vi "Host_AutoApproach(Original).vi"() -> ()   [LabVIEW 2014]
uses:
  <vilib>/userdefined/High Color/nirio_resource_hc.ctl
  <vilib>/Instr/_visa.llb/VISA Configure Serial Port (Instr).vi
  <vilib>/FPGAPlugInAG/PCIe-7851R/niLvFpga_Open_PCIe-7851R.vi
  <vilib>/rvi/interface/common/dynamic/niFpgaDynamicAddResources.vi
  <vilib>/FPGAPlugInAG/Dynamic/niLvFpga_Run_Dynamic.vi
  <vilib>/Utility/error.llb/Error Cluster From Error Code.vi
  <vilib>/rvi/errors/niLvFpgaAdjustHostInterfaceError.vi
  <vilib>/FPGAPlugInAG/Dynamic/niLvFpga_Close_Dynamic.vi
  <vilib>/rvi/interface/nirviOpenFPGA/nirviOpenFPGA.xnode
  XZFPGAWithinHopping(Original)/FPGA Bitfiles/XZFPGAWithinHopp_FPGATarget_ApproachingStep(_p7iJPTKslXo.lvbitx
  <vilib>/rvi/interface/nirviMethod/nirviMethod.xnode
  <vilib>/rvi/interface/nirviReadWriteControl/nirviReadWriteControl.xnode
  <vilib>/rvi/interface/nirviCloseFPGA/nirviCloseFPGA.xnode
  NiFpgaLv.dll
  <vilib>/rvi/interface/Simulation/niFpgaSimulationCallBeginRW.vi
panel:
  out "ZCalPos":i32
  in  "PIZ":T1
  in  "ContinuousReapproach":bool
  in  "UseMemoryPos?":bool=TRUE
  out "ZRealPos":i16
  out "Curr":i16
  out "PIZPosDia":i16(graph)
  out "CurrDia":i16(graph)
  in  "stop":bool
  out "RoughZPos?":dbl
  out "Error?":string
  in  "RoughZ":refnum<visa-resource-name>
  in  "RoughZInitPos":dbl format="%#_13g"
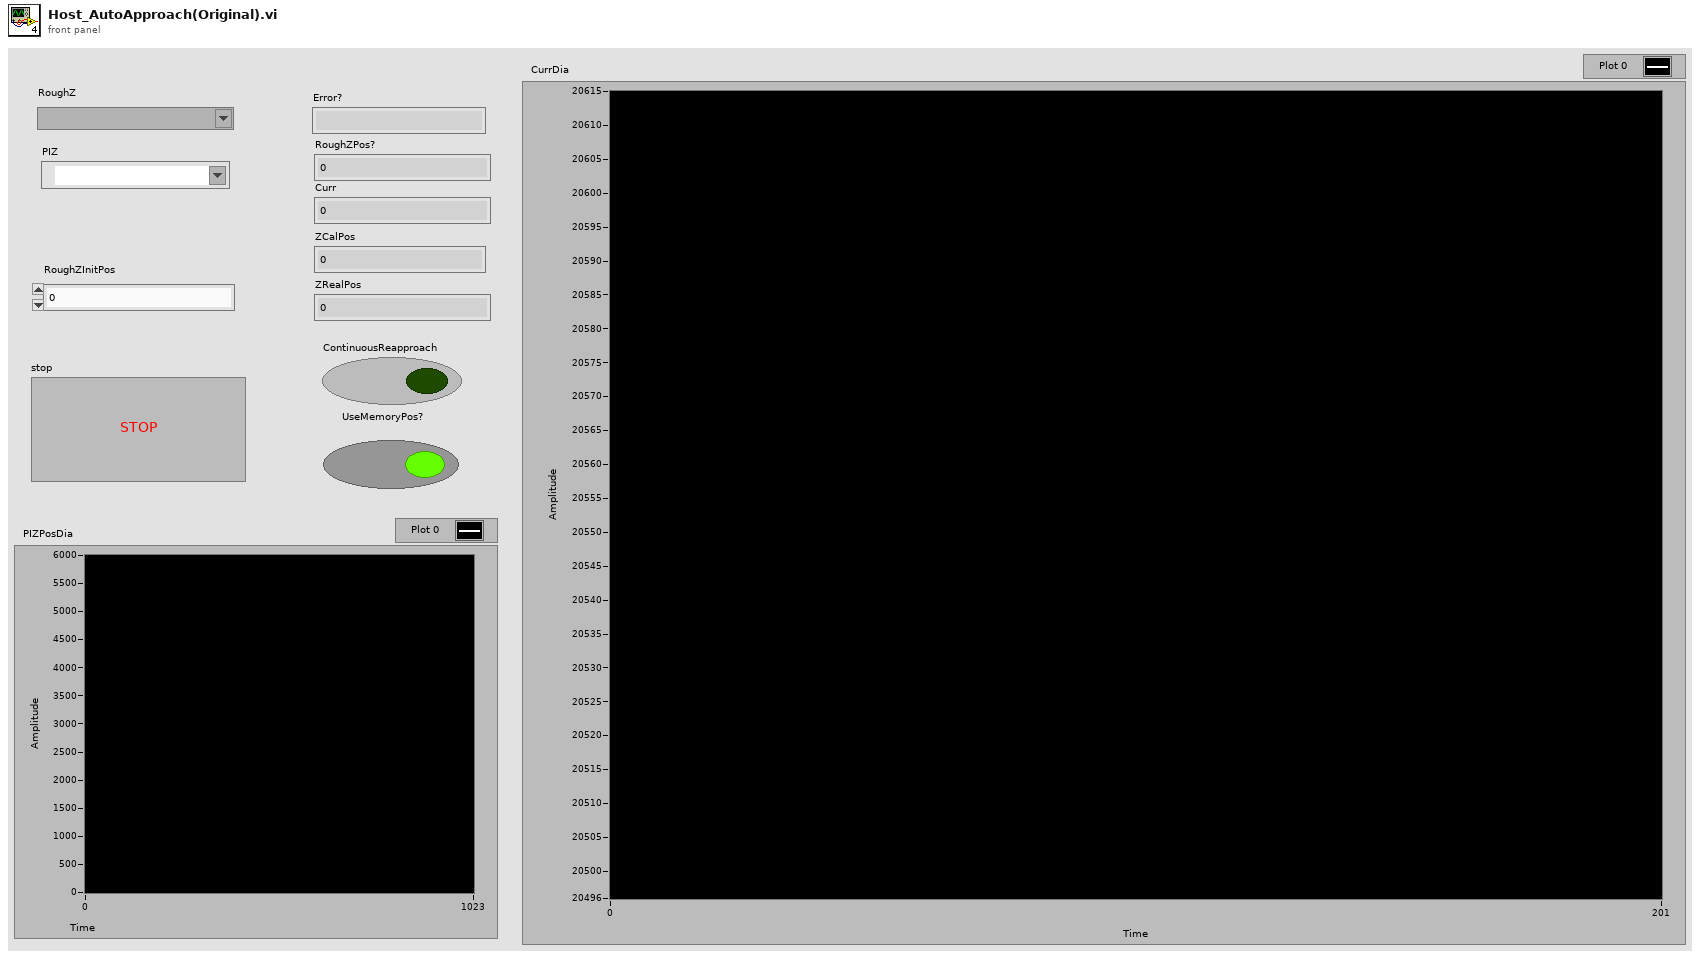
[diagram p1: front panel]
types:
  T1 = typedef "nirio_resource_hc.ctl" = tag
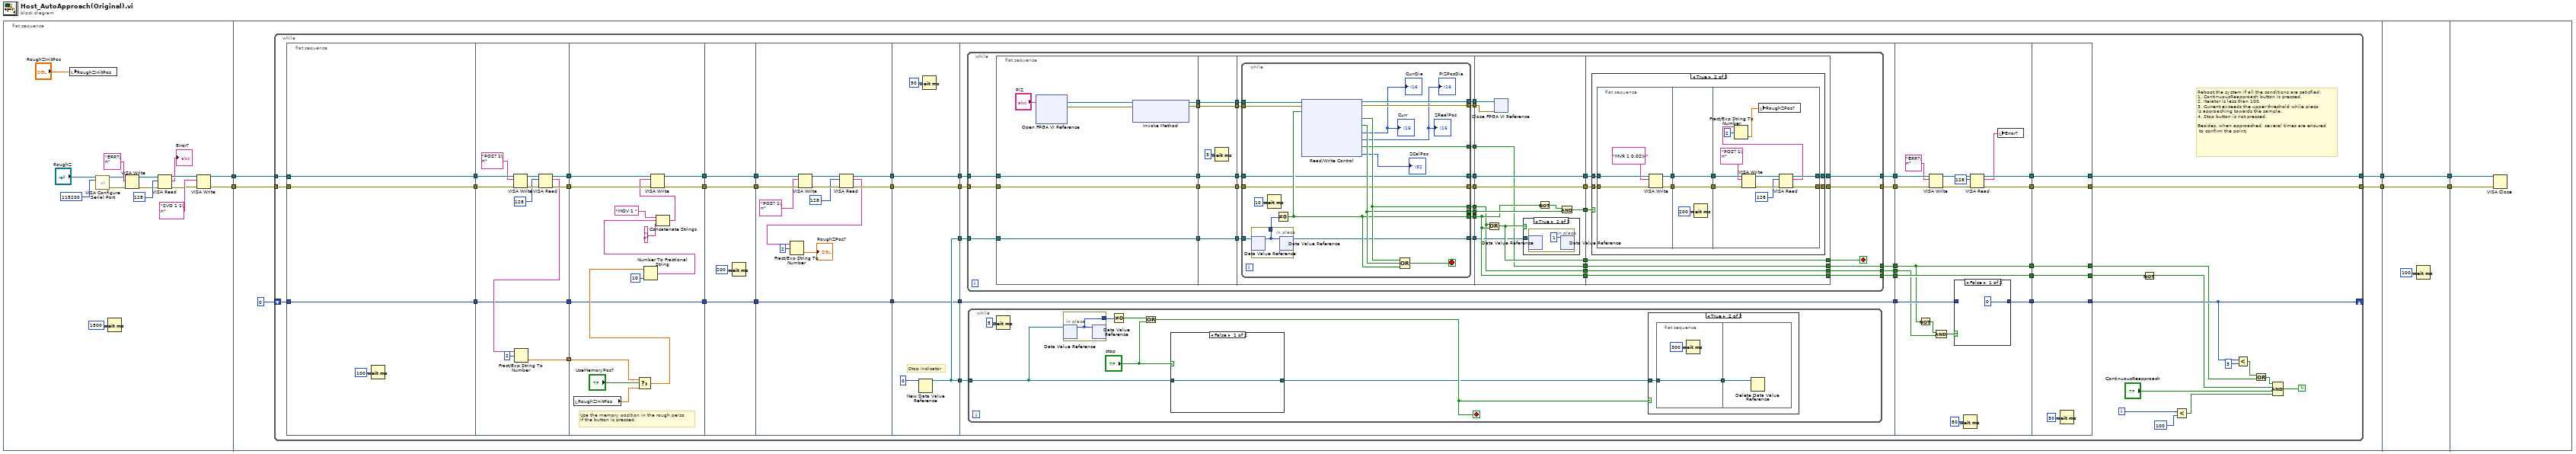
[diagram p0: block diagram]
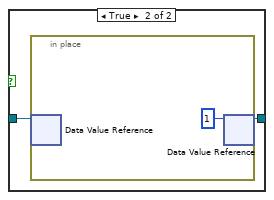
[diagram p3: hidden frame]
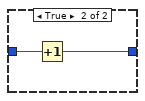
[diagram p6: hidden frame]
diagram:
  n1 = flat-sequence {
    tunnel: [w8] -> w2
    tunnel: [w7] -> w1
    tunnel: [w26] -> w5
    tunnel: [w25] -> w3
    tunnel: w2 -> [w24]
    tunnel: w1 -> [w23]
    tunnel: [w318] -> w6
    tunnel: w5 -> [w318]
    tunnel: [w317] -> w4
    tunnel: w3 -> [w317]
    tunnel: w6 -> [w320]
    tunnel: w4 -> [w319]
    frame #0 {
      n2 = local write "RoughZInitPos"("RoughZInitPos") -> ()
      n3 = call-poly "VISA Configure Serial Port"("VISA resource name"="RoughZ", "baud rate (9600)"=u32 115200) -> ("VISA resource name out"=w11:refnum<visa-resource-name>, "error out"=w12:errorcluster)  [unwired: 12 in]
      n4 = Wait (ms)(milliseconds to wait=u32 1500) -> ()  [unwired: 1 out]
      n5 = VISA Write(VISA resource name=w11, write buffer="ERR?\n", error in (no error)=w12) -> (VISA resource name out=w14:refnum<visa-resource-name>, error out=w15:errorcluster)  [unwired: 1 out]
      n6 = VISA Read(VISA resource name=w14, byte count=u32 128, error in (no error)=w15) -> (VISA resource name out=w18:refnum<visa-resource-name>, read buffer=→"Error?":string, error out=w19:errorcluster)  [unwired: 1 out]
      n7 = VISA Write(VISA resource name=w18, write buffer="SVO 1 1\n", error in (no error)=w19) -> (VISA resource name out=w8:refnum<visa-resource-name>, error out=w7:errorcluster)  [unwired: 1 out]
    }
    frame #1 {
      n8 = while {
        shift-right: [w36] -> _
        shift-left: 0 -> [w46]
        tunnel: [w31] -> w26
        tunnel: [w30] -> w25
        tunnel: w24 -> [w29]
        tunnel: w23 -> [w28]
        i -> [w57]
        stop <- w51 continue-if-true
        # "Reboot the system if all the conditions are satisfied:\n1. ContinuousReapproach button is pressed.\n2. Iterator is less than 100.\n3. Current exceeds the upper threshold while piezo\nis approaching towards the sample.\n4. Stop button is not pressed.\n\nBesides, when approached, several times are ensured\n to confirm the point."
        n9 = flat-sequence {
          tunnel: [w78] -> w76
          tunnel: [w77] -> w75
          tunnel: w46 -> [w80]
          tunnel: [w80] -> w45
          tunnel: w29 -> [w78]
          tunnel: w28 -> [w77]
          tunnel: w76 -> [w92]
          tunnel: [w88] -> w74
          tunnel: w75 -> [w91]
          tunnel: [w87] -> w73
          tunnel: [w82] -> w72
          tunnel: w45 -> [w81]
          tunnel: [w81] -> w44
          tunnel: w74 -> [w106]
          tunnel: w73 -> [w105]
          tunnel: [w99] -> w71
          tunnel: [w98] -> w70
          tunnel: w72 -> [w96]
          tunnel: w44 -> [w93]
          tunnel: [w93] -> w41
          tunnel: w71 -> [w110]
          tunnel: w70 -> [w109]
          tunnel: [w110] -> w69
          tunnel: [w109] -> w68
          tunnel: [w107] -> w42
          tunnel: w41 -> [w107]
          tunnel: w69 -> [w122]
          tunnel: w68 -> [w121]
          tunnel: [w116] -> w67
          tunnel: [w115] -> w66
          tunnel: [w111] -> w43
          tunnel: w42 -> [w111]
          tunnel: [w128] -> w65
          tunnel: [w127] -> w64
          tunnel: [w124] -> w63
          tunnel: [w124] -> w62
          tunnel: w66 -> [w127]
          tunnel: w67 -> [w128]
          tunnel: w43 -> [w123]
          tunnel: [w123] -> w40
          tunnel: w65 -> [w138]
          tunnel: w64 -> [w137]
          tunnel: w63 -> [w136]
          tunnel: w62 -> [w135]
          tunnel: [w134] -> w61
          tunnel: [w133] -> w60
          tunnel: [w132] -> w55
          tunnel: [w131] -> w50
          tunnel: w40 -> [w130]
          tunnel: [w130] -> w39
          tunnel: [w129] -> w38
          tunnel: w61 -> [w306]
          tunnel: w60 -> [w305]
          tunnel: [w300] -> w59
          tunnel: [w299] -> w58
          tunnel: w55 -> [w295]
          tunnel: [w295] -> w54
          tunnel: w50 -> [w292]
          tunnel: [w292] -> w49
          tunnel: w39 -> [w296]
          tunnel: w38 -> [w290]
          tunnel: [w293] -> w37
          tunnel: [w314] -> w48
          tunnel: [w313] -> w33
          tunnel: [w312] -> w31
          tunnel: [w311] -> w30
          tunnel: w49 -> [w313]
          tunnel: w54 -> [w314]
          tunnel: w58 -> [w311]
          tunnel: w59 -> [w312]
          tunnel: w37 -> [w310]
          tunnel: [w310] -> w36
          frame #0 {
            n10 = Wait (ms)(milliseconds to wait=u32 100) -> ()  [unwired: 1 out]
          }
          frame #1 {
            n11 = VISA Write(VISA resource name=w92, write buffer="POS? 1\n", error in (no error)=w91) -> (VISA resource name out=w90:refnum<visa-resource-name>, error out=w89:errorcluster)  [unwired: 1 out]
            n12 = VISA Read(VISA resource name=w90, byte count=u32 128, error in (no error)=w89) -> (VISA resource name out=w88:refnum<visa-resource-name>, read buffer=w84:string, error out=w87:errorcluster)  [unwired: 1 out]
            n13 = Fract/Exp String To Number(string=w84, offset=2) -> (number=w82:dbl)  [unwired: 2 in, 1 out]
          }
          frame #2 {
            # "Use the memory position in the rough peizo\nif the button is pressed."
            n14 = local read "RoughZInitPos"() -> (w95:dbl)
            n15 = Select(t=w96, s="UseMemoryPos?", f=w95) -> (s? t:f=w94:dbl)
            n16 = Number To Fractional String(number=w94, precision (6)=i16 10) -> (F-format string=w102:string)  [unwired: 2 in]
            n17 = Concatenate Strings("MOV 1 " ("string"), w102, "\n" ("string")) -> (w104:string)
            n18 = VISA Write(VISA resource name=w106, write buffer=w104, error in (no error)=w105) -> (VISA resource name out=w99:refnum<visa-resource-name>, error out=w98:errorcluster)  [unwired: 1 out]
          }
          frame #3 {
            n19 = Wait (ms)(milliseconds to wait=u32 200) -> ()  [unwired: 1 out]
          }
          frame #4 {
            n20 = VISA Write(VISA resource name=w122, write buffer="POS? 1\n", error in (no error)=w121) -> (VISA resource name out=w119:refnum<visa-resource-name>, error out=w118:errorcluster)  [unwired: 1 out]
            n21 = VISA Read(VISA resource name=w119, byte count=u32 128, error in (no error)=w118) -> (VISA resource name out=w116:refnum<visa-resource-name>, read buffer=w114:string, error out=w115:errorcluster)  [unwired: 1 out]
            n22 = Fract/Exp String To Number(string=w114, offset=2) -> (number=→"RoughZPos?":dbl)  [unwired: 2 in, 1 out]
          }
          frame #5 {
            # "Stop indicator"
            n23 = New Data Value Reference(data value=0) -> (data value reference=w124:refnum<data-value>)  [unwired: 1 in, 1 out]
            n24 = Wait (ms)(milliseconds to wait=u32 50) -> ()  [unwired: 1 out]
          }
          frame #6 {
            n25 = while {
              tunnel: w138 -> [w190]
              tunnel: w137 -> [w189]
              tunnel: w135 -> [w188]
              tunnel: [w174] -> w134
              tunnel: [w173] -> w133
              tunnel: [w171] -> w132
              tunnel: [w168] -> w131
              tunnel: [w156] -> w129
              stop <- w175 stop-if-true
              n26 = flat-sequence {
                tunnel: w190 -> [w195]
                tunnel: w189 -> [w194]
                tunnel: [w198] -> w167
                tunnel: [w197] -> w165
                tunnel: [w196] -> w163
                tunnel: w188 -> [w196]
                tunnel: [w195] -> w161
                tunnel: [w194] -> w159
                tunnel: w167 -> [w204]
                tunnel: [w204] -> w166
                tunnel: w165 -> [w203]
                tunnel: [w203] -> w164
                tunnel: w163 -> [w202]
                tunnel: [w202] -> w162
                tunnel: w161 -> [w201]
                tunnel: [w201] -> w160
                tunnel: w159 -> [w200]
                tunnel: [w200] -> w158
                tunnel: w166 -> [w218]
                tunnel: w164 -> [w217]
                tunnel: w162 -> [w216]
                tunnel: w160 -> [w215]
                tunnel: w158 -> [w214]
                tunnel: [w213] -> w187
                tunnel: [w212] -> w186
                tunnel: [w211] -> w185
                tunnel: [w210] -> w184
                tunnel: [w209] -> w183
                tunnel: [w208] -> w182
                tunnel: [w207] -> w181
                tunnel: [w206] -> w180
                tunnel: [w205] -> w170
                tunnel: w187 -> [w238]
                tunnel: w186 -> [w246]
                tunnel: w185 -> [w241]
                tunnel: w184 -> [w249]
                tunnel: w183 -> [w248]
                tunnel: w182 -> [w243]
                tunnel: w181 -> [w244]
                tunnel: w180 -> [w239]
                tunnel: [w245] -> w179
                tunnel: [w244] -> w178
                tunnel: [w243] -> w177
                tunnel: [w242] -> w176
                tunnel: [w241] -> w172
                tunnel: w170 -> [w240]
                tunnel: [w240] -> w169
                tunnel: [w238] -> w157
                tunnel: w179 -> [w260]
                tunnel: w178 -> [w259]
                tunnel: w177 -> [w258]
                tunnel: w176 -> [w257]
                tunnel: [w257] -> w175
                tunnel: [w256] -> w174
                tunnel: [w255] -> w173
                tunnel: w172 -> [w254]
                tunnel: [w254] -> w171
                tunnel: w169 -> [w253]
                tunnel: [w253] -> w168
                tunnel: w157 -> [w252]
                tunnel: [w252] -> w156
                frame #0 {
                  n27 = xnode "Open FPGA VI Reference"("resource name"="PIZ") -> ("FPGA VI Reference Out"=w193:refnum<k20>, "error out"=w192:errorcluster)  [unwired: 1 in]
                  n28 = xnode "Invoke Method"("FPGA VI Reference In"=w193, "error in"=w192) -> ("FPGA VI Reference Out"=w198:refnum<k20>, "error out"=w197:errorcluster)  [unwired: 1 in]
                }
                frame #1 {
                  n29 = Wait (ms)(milliseconds to wait=u32 3) -> ()  [unwired: 1 out]
                }
                frame #2 {
                  n30 = while {
                    tunnel: w218 -> [w236]
                    tunnel: w217 -> [w235]
                    tunnel: w216 -> [w234]
                    tunnel: w215 -> [w226]
                    tunnel: w214 -> [w225]
                    tunnel: [w231] -> w213
                    tunnel: [w230] -> w212
                    tunnel: [w229] -> w211
                    tunnel: [w228] -> w210
                    tunnel: [w227] -> w209
                    tunnel: [w226] -> w207
                    tunnel: [w225] -> w208
                    tunnel: [w224] -> w206
                    tunnel: [w221] -> w205
                    stop <- w232 stop-if-true
                    n31 = in-place {
                      in-place-border: [w237] -> w233
                      n32 = in-place-dvr #1(w234) -> (w237:i32)  [unwired: 1 out]
                      n33 = in-place-dvr #1(w237) -> (w224:refnum<data-value>)  [unwired: 1 out]
                    }
                    n34 = Wait (ms)(milliseconds to wait=u32 10) -> ()  [unwired: 1 out]
                    n35 = Not Equal To 0?(x=w233) -> (x != 0?=w229:bool)
                    n36 = xnode "Read/Write Control"("FPGA VI Reference In"=w236, "error in"=w235, "stop"=w229) -> ("FPGA VI Reference Out"=w228:refnum<k20>, "error out"=w227:errorcluster, "Approached?"=w231:bool, "PIZRangeExceeded?"=w230:bool, "PresCurr"=→"CurrDia" →"Curr":i16, "RealPIZPos"=→"PIZPosDia" →"ZRealPos":i16, "ExceedUpperLimit?"=w221:bool, "ZCalPos"=→"ZCalPos":i32)
                    n37 = Compound Arithmetic op=OR(w231, w230, w229) -> (w232:bool)
                  }
                }
                frame #3 {
                  n38 = Or(x=w238, y=w241) -> (x .or. y?=w242:bool)
                  n39 = xnode "Close FPGA VI Reference"("FPGA VI Reference In"=w249, "error in"=w248) -> ()  [unwired: 1 out]
                  n40 = case shown="True" w242 {
                    tunnel: w239 -> [_ w250]
                    frame False {
                    }
                    frame True {
                      n41 = in-place {
                        n42 = in-place-dvr #2(w250) -> ()  [unwired: 2 out]
                        n43 = in-place-dvr #2(1 ("data value")) -> ()  [unwired: 2 out]
                      }
                    }
                  }
                  n44 = Not(x=w241) -> (.not. x?=w247:bool)
                  n45 = And(x=w247, y=w246) -> (x .and. y?=w245:bool)
                }
                frame #4 {
                  n46 = case shown="True" w260 {
                    tunnel: w259 -> [w262 w270]
                    tunnel: w258 -> [w261 w269]
                    tunnel: [w262 w264] -> w256
                    tunnel: [w261 w263] -> w255
                    frame False {
                    }
                    frame True {
                      n47 = flat-sequence {
                        tunnel: w270 -> [w275]
                        tunnel: w269 -> [w274]
                        tunnel: [w272] -> w268
                        tunnel: [w271] -> w267
                        tunnel: w268 -> [w278]
                        tunnel: w267 -> [w277]
                        tunnel: [w278] -> w266
                        tunnel: [w277] -> w265
                        tunnel: w266 -> [w289]
                        tunnel: w265 -> [w288]
                        tunnel: [w283] -> w264
                        tunnel: [w282] -> w263
                        frame #0 {
                          n48 = VISA Write(VISA resource name=w275, write buffer="MVR 1 0.02\n", error in (no error)=w274) -> (VISA resource name out=w272:refnum<visa-resource-name>, error out=w271:errorcluster)  [unwired: 1 out]
                        }
                        frame #1 {
                          n49 = Wait (ms)(milliseconds to wait=u32 200) -> ()  [unwired: 1 out]
                        }
                        frame #2 {
                          n50 = VISA Write(VISA resource name=w289, write buffer="POS? 1\n", error in (no error)=w288) -> (VISA resource name out=w286:refnum<visa-resource-name>, error out=w285:errorcluster)  [unwired: 1 out]
                          n51 = VISA Read(VISA resource name=w286, byte count=u32 128, error in (no error)=w285) -> (VISA resource name out=w283:refnum<visa-resource-name>, read buffer=w281:string, error out=w282:errorcluster)  [unwired: 1 out]
                          n52 = Fract/Exp String To Number(string=w281, offset=2) -> (number=w279:dbl)  [unwired: 2 in, 1 out]
                          n53 = local write "RoughZPos?"(w279) -> ()
                        }
                      }
                    }
                  }
                }
              }
            }
            n54 = while {
              tunnel: w136 -> [w144]
              stop <- w140 stop-if-true
              n55 = Wait (ms)(milliseconds to wait=u32 5) -> ()  [unwired: 1 out]
              n56 = in-place {
                in-place-border: [w151] -> w143
                n57 = in-place-dvr #3(w144) -> (w151:i32)  [unwired: 1 out]
                n58 = in-place-dvr #3(w151) -> ()  [unwired: 2 out]
              }
              n59 = Not Equal To 0?(x=w143) -> (x != 0?=w142:bool)
              n60 = Or(x=w142, y="stop") -> (x .or. y?=w140:bool)
              n61 = case shown="False" "stop" {
                tunnel: w144 -> [w152 w154]
                tunnel: [w152 w153] -> w139
                frame False {
                }
                frame True {
                  n62 = in-place {
                    n63 = in-place-dvr #4(w154) -> ()  [unwired: 2 out]
                    n64 = in-place-dvr #4(1 ("data value")) -> (w153:refnum<data-value>)  [unwired: 1 out]
                  }
                }
              }
              n65 = case shown="True" w140 {
                tunnel: w139 -> [_ w147]
                frame False {
                }
                frame True {
                  n66 = flat-sequence {
                    tunnel: w147 -> [w148]
                    tunnel: [w148] -> w146
                    tunnel: w146 -> [w150]
                    frame #0 {
                      n67 = Wait (ms)(milliseconds to wait=u32 300) -> ()  [unwired: 1 out]
                    }
                    frame #1 {
                      n68 = Delete Data Value Reference(data value reference=w150) -> ()  [unwired: 1 in, 2 out]
                    }
                  }
                }
              }
            }
          }
          frame #7 {
            n69 = Not(x=w292) -> (.not. x?=w291:bool)
            n70 = VISA Write(VISA resource name=w306, write buffer="ERR?\n", error in (no error)=w305) -> (VISA resource name out=w304:refnum<visa-resource-name>, error out=w303:errorcluster)  [unwired: 1 out]
            n71 = Compound Arithmetic op=AND(w291, w290) -> (w294:bool)
            n72 = case shown="False" w294 {
              tunnel: w296 -> [_ w309]
              tunnel: [0 w308] -> w293
              frame False {
              }
              frame True {
                n73 = Increment(x=w309) -> (x+1=w308:i32)
              }
            }
            n74 = Wait (ms)(milliseconds to wait=u32 50) -> ()  [unwired: 1 out]
            n75 = VISA Read(VISA resource name=w304, byte count=u32 128, error in (no error)=w303) -> (VISA resource name out=w300:refnum<visa-resource-name>, read buffer=w298:string, error out=w299:errorcluster)  [unwired: 1 out]
            n76 = local write "Error?"(w298) -> ()
          }
          frame #8 {
            n77 = Wait (ms)(milliseconds to wait=u32 50) -> ()  [unwired: 1 out]
          }
        }
        n78 = Not(x=w48) -> (.not. x?=w47:bool)
        n79 = Less?(x=w57, y=100) -> (x < y?=w52:bool)
        n80 = Less?(x=w36, y=3) -> (x < y?=w34:bool)
        n81 = Or(x=w34, y=w33) -> (x .or. y?=w32:bool)
        n82 = Compound Arithmetic op=AND(w32, w47, "ContinuousReapproach", w52) -> (w51:bool)
      }
    }
    frame #2 {
      n83 = Wait (ms)(milliseconds to wait=u32 100) -> ()  [unwired: 1 out]
    }
    frame #3 {
      n84 = VISA Close(VISA resource name=w320, error in (no error)=w319) -> ()  [unwired: 1 out]
    }
  }
